vi "LeerBaseDatos.vi"(8 "error in (no error)":errorcluster, 11 "Prueba01 in":refnum<class "Prueba01.lvclass">) -> (0 "error out":errorcluster, 3 "Prueba01 out":refnum<class "Prueba01.lvclass">)   [LabVIEW 2019, in "Prueba01.lvclass"]
uses:
  Prueba01.lvclass
  Controles/BD_P01.ctl
  Prueba01.lvclass/Prueba01.ctl
  Base de Datos/SQLiteConnector/SQLiteConnection.lvclass
  Base de Datos/Base de Datos.lvclass
panel:
  out "BD":T1
  in  "Tipo Equipo":enum16{"Sonometro", "Calibrador", "Dosimetro"}(ring)
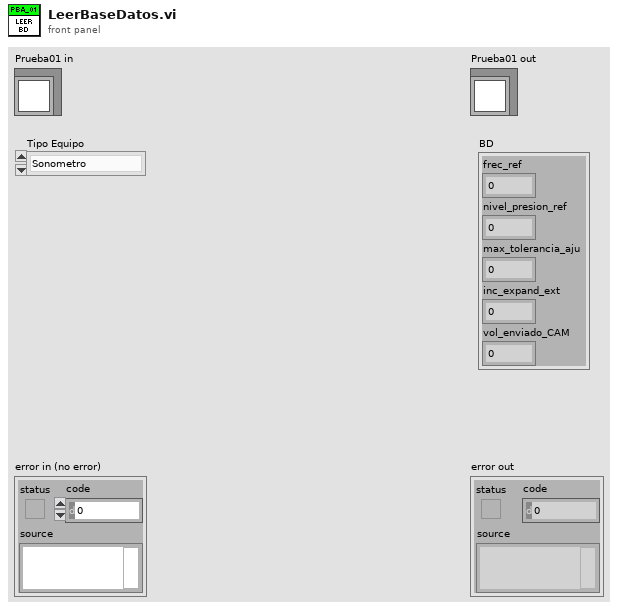
[diagram p1: front panel]
types:
  T1 = typedef "Prueba01.lvclass/BD_P01.ctl" = cluster{"frec_ref":dbl, "nivel_presion_ref":dbl, "max_tolerancia_aju":dbl, "inc_expand_ext":dbl, "vol_enviado_CAM":dbl}
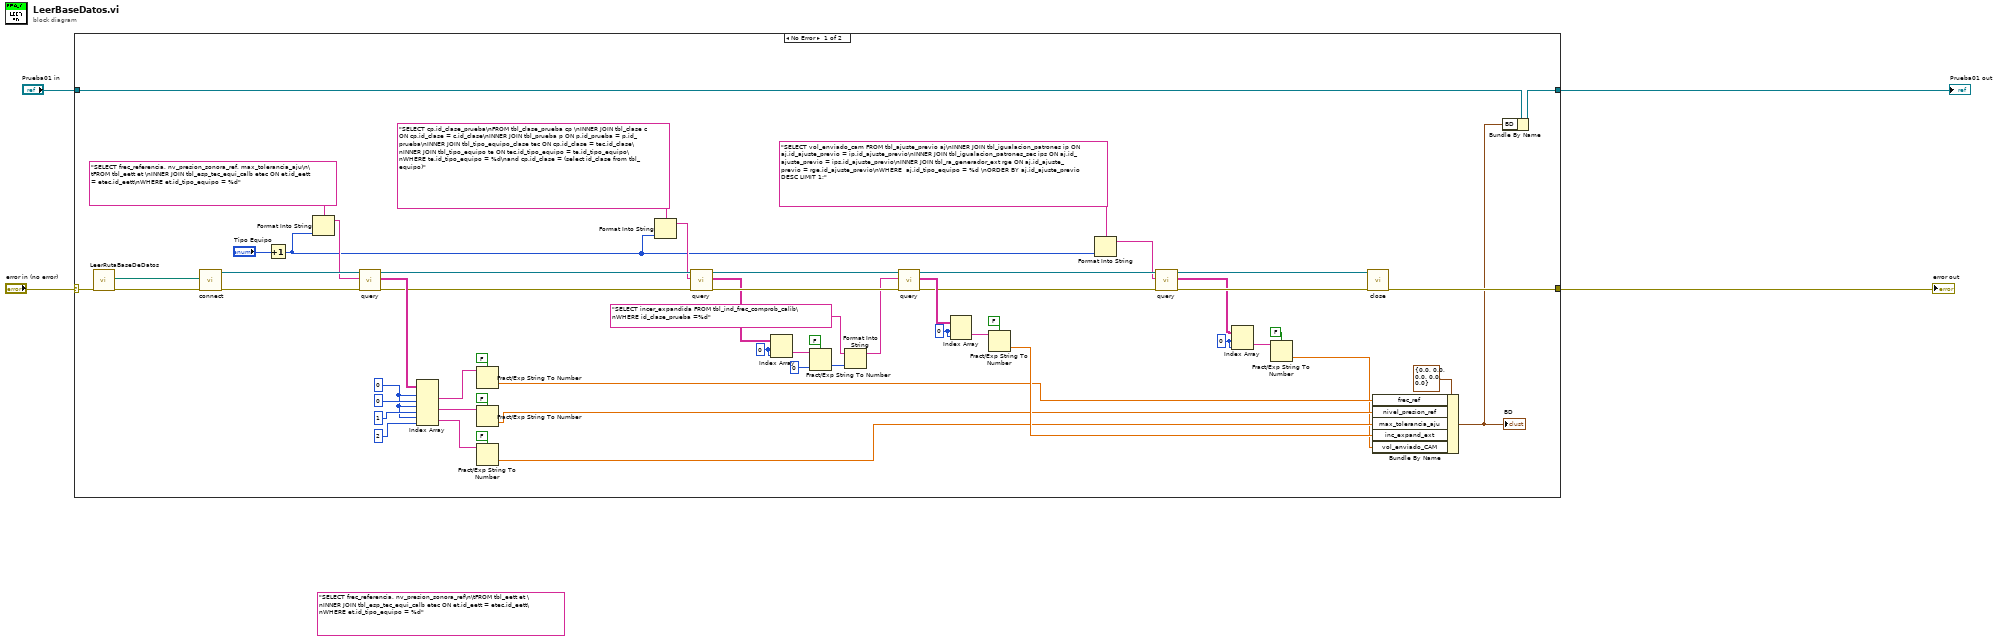
[diagram p0: block diagram]
diagram:
  (unwired) "SELECT frec_referencia, nv_presion_sonora_ref\n\tFROM tbl_eett et \nINNER JOIN tbl_esp_tec_equi_calb etec ON et.id_eett = etec.id_eett\nWHERE et.id_tipo_equipo = %d" ("format string")
  n1 = case shown="No Error" "error in (no error)" {
    selector: "error in (no error)" -> [w61 w64]
    tunnel: [w53 w64] -> w3
    tunnel: [w18 w63] -> w1
    tunnel: "Prueba01 in" -> [w62 w63]
    frame No Error {
      w9 = 0 ("index (row)")
      w25 = 0 ("index (row)")
      w36 = 0 ("index (row)")
      w45 = 0 ("index (row)")
      n2 = call "LeerRutaBaseDeDatos.vi"("error in (no error)"=w61) -> ("error out"=w55:errorcluster, "Database Path"=w54:path)  [unwired: 9 in]
      n3 = call "connect.vi"("error in (no error)"=w55, "Database Path"=w54) -> ("error out"=w57:errorcluster, "object out"=w58:refnum<class "SQLiteConnection.lvclass">)  [unwired: 8 in]
      n4 = Increment(x="Tipo Equipo") -> (x+1=w10:enum16{"Sonometro", "Calibrador", "Dosimetro"})
      n5 = Format Into String(format string="SELECT frec_referencia, nv_presion_sonora_ref, max_tolerancia_aju\n\tFROM tbl_eett et \nINNER JOIN tbl_esp_tec_equi_calb etec ON et.id_eett = etec.id_eett\nWHERE et.id_tipo_equipo = %d", w10) -> (resulting string=w56:string)  [unwired: 2 in, 1 out]
      n6 = call "query.vi"("error in (no error)"=w57, "SQL Statement"=w56, "object in"=w58) -> ("error out"=w41:errorcluster, "result"=w52:string[][], "object out"=w40:refnum<class "SQLiteConnection.lvclass">)  [unwired: 5 in, 1 out]
      n7 = Index Array(array=w52, index (row) #1=w45, index (col) #1=0 ("disabled index (col)"), index (row) #2=w45, index (col) #2=1 ("disabled index (col)"), index (row) #3=w45, index (col) #3=2 ("index (col)")) -> (element #1=w49:string, element #2=w48:string, element #3=w43:string)
      n8 = Fract/Exp String To Number(use system decimal point (T)=FALSE, string=w49) -> (number=w21:dbl)  [unwired: 2 in, 1 out]
      n9 = Fract/Exp String To Number(use system decimal point (T)=FALSE, string=w48) -> (number=w20:dbl)  [unwired: 2 in, 1 out]
      n10 = Fract/Exp String To Number(use system decimal point (T)=FALSE, string=w43) -> (number=w19:dbl)  [unwired: 2 in, 1 out]
      n11 = Format Into String(format string="SELECT cp.id_clase_prueba\nFROM tbl_clase_prueba cp \nINNER JOIN tbl_clase c ON cp.id_clase = c.id_clase\nINNER JOIN tbl_prueba p ON p.id_prueba = p.id_prueba\nINNER JOIN tbl_tipo_equipo_clase tec ON cp.id_clase = tec.id_clase\nINNER JOIN tbl_tipo_equipo te ON tec.id_tipo_equipo = te.id_tipo_equipo\nWHERE te.id_tipo_equipo = %d\nand cp.id_clase = (select id_clase from tbl_equipo)", w10) -> (resulting string=w38:string)  [unwired: 2 in, 1 out]
      n12 = call "query.vi"("error in (no error)"=w41, "SQL Statement"=w38, "object in"=w40) -> ("error out"=w37:errorcluster, "result"=w35:string[][], "object out"=w28:refnum<class "SQLiteConnection.lvclass">)  [unwired: 5 in, 1 out]
      n13 = Index Array(array=w35, index (row)=w36, index (col)=w36) -> (element=w33:string)
      n14 = Fract/Exp String To Number(use system decimal point (T)=FALSE, string=w33, default (0 dbl)=0 ("index (row)")) -> (number=w32:i32)  [unwired: 1 in, 1 out]
      n15 = Format Into String(format string="SELECT incer_expandida FROM tbl_ind_frec_comprob_calib\nWHERE id_clase_prueba =%d", w32) -> (resulting string=w29:string)  [unwired: 2 in, 1 out]
      n16 = call "query.vi"("error in (no error)"=w37, "SQL Statement"=w29, "object in"=w28) -> ("error out"=w15:errorcluster, "result"=w24:string[][], "object out"=w16:refnum<class "SQLiteConnection.lvclass">)  [unwired: 5 in, 1 out]
      n17 = Index Array(array=w24, index (row)=w25, index (col)=w25) -> (element=w27:string)
      n18 = Fract/Exp String To Number(use system decimal point (T)=FALSE, string=w27) -> (number=w22:dbl)  [unwired: 2 in, 1 out]
      n19 = Format Into String(format string="SELECT vol_enviado_cam FROM tbl_ajuste_previo aj\nINNER JOIN tbl_igualacion_patrones ip ON aj.id_ajuste_previo = ip.id_ajuste_previo\nINNER JOIN tbl_igualacion_patrones_sec ips ON aj.id_ajuste_previo = ips.id_ajuste_previo\nINNER JOIN tbl_ra_generador_ext rge ON aj.id_ajuste_previo = rge.id_ajuste_previo\nWHERE  aj.id_tipo_equipo = %d \nORDER BY aj.id_ajuste_previo DESC LIMIT 1;", w10) -> (resulting string=w11:string)  [unwired: 2 in, 1 out]
      n20 = call "query.vi"("error in (no error)"=w15, "SQL Statement"=w11, "object in"=w16) -> ("error out"=w13:errorcluster, "result"=w6:string[][], "object out"=w14:refnum<class "SQLiteConnection.lvclass">)  [unwired: 5 in, 1 out]
      n21 = Index Array(array=w6, index (row)=w9, index (col)=w9) -> (element=w7:string)
      n22 = Fract/Exp String To Number(use system decimal point (T)=FALSE, string=w7) -> (number=w5:dbl)  [unwired: 2 in, 1 out]
      n23 = call-dynamic "close.vi"("error in (no error)"=w13, "object in"=w14) -> ("error out"=w53:errorcluster)  [unwired: 8 in, 1 out]
      n24 = Bundle By Name(cluster=T1 {"frec_ref"=0.0, "nivel_presion_ref"=0.0, "max_tolerancia_aju"=0.0, "inc_expand_ext"=0.0, "vol_enviado_CAM"=0.0}, "frec_ref"=w21, "nivel_presion_ref"=w20, "max_tolerancia_aju"=w19, "inc_expand_ext"=w22, "vol_enviado_CAM"=w5) -> (w17:T1)
      "BD" <- w17
      n25 = Bundle By Name(cluster=w62, "BD"=w17) -> (w18:refnum<class "Prueba01.lvclass">)
    }
    frame Error {
    }
  }
  "error out" <- w3
  "Prueba01 out" <- w1
